vi "add_percentage_for_floating_datatype.vi"(8 "error in (no error)":errorcluster, 11 "String In":string) -> (0 "error out":errorcluster, 3 "String Out":string)   [LabVIEW 2018]
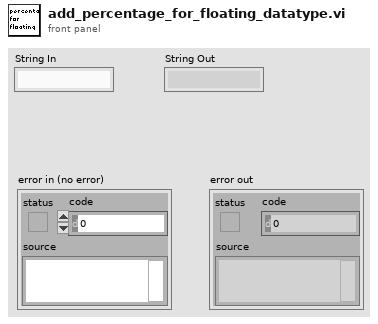
[diagram p1: front panel]
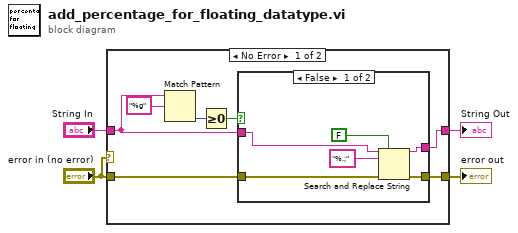
[diagram p0: block diagram]
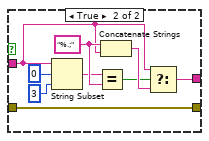
[diagram p2: hidden frame]
diagram:
  n1 = case shown="No Error" "error in (no error)" {
    selector: "error in (no error)" -> [_ w28]
    tunnel: [w11 w27] -> w4
    tunnel: "String In" -> [w8 w27]
    tunnel: "error in (no error)" -> [w6 _]
    tunnel: [w5 w28] -> w2
    frame No Error {
      n2 = Match Pattern(string=w8, regular expression="%g") -> (offset past match=w9:i32)  [unwired: 4 out]
      n3 = Greater Or Equal To 0?(x=w9) -> (x >= 0?=w7:bool)
      n4 = case shown="False" w7 {
        tunnel: [w15 w26] -> w11
        tunnel: w8 -> [w17 w19]
        tunnel: w6 -> [w13 w18]
        tunnel: [w12 w18] -> w5
        frame False {
          n5 = Search and Replace String(replace all?=FALSE ("replace all? (F)"), input string=w17, search string="%.;", error in=w13) -> (result string=w15:string, error out=w12:errorcluster)  [unwired: 6 out]
        }
        frame True {
          w24 = "%.;"
          n6 = String Subset(string=w19, offset (0)=0, length (rest)=3 ("length (rest)")) -> (substring=w22:string)
          n7 = Equal?(x=w22, y=w24) -> (x = y?=w23:bool)
          n8 = Concatenate Strings(w24, w19) -> (w25:string)
          n9 = Select(t=w19, s=w23, f=w25) -> (s? t:f=w26:string)
        }
      }
    }
    frame Error {
    }
  }
  "String Out" <- w4
  "error out" <- w2
